vi "GetSettings.vi"(8 "error in (no error)":errorcluster, 10 "SettingsToRetrieve":variant, 11 "NHRDCPower in":refnum<class "NHRDCPower.lvclass">) -> (0 "error out":errorcluster, 1 "DeviceConfig&Meas":variant, 2 "RetrievedSettings":variant, 3 "NHRDCPower Out":refnum<class "NHRDCPower.lvclass">)   [LabVIEW 2018, in "AcPwrPlugins.lvlib" / "NHRDCPower.lvclass"]
doc: "This VI retrieves the configuration or measurement settings."
uses:
  NHRDCPower.lvclass
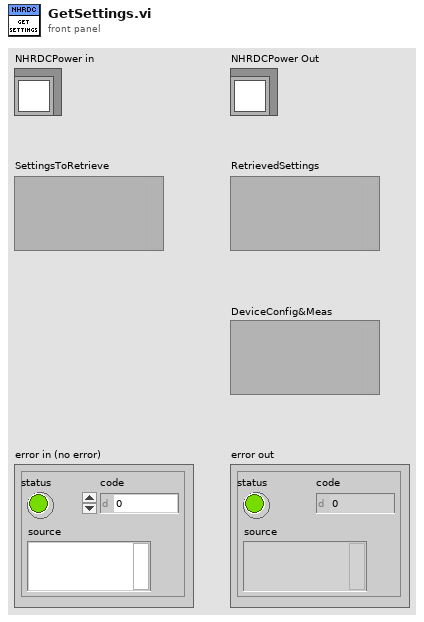
[diagram p1: front panel]
types:
  T1 = typedef "AcPwrPlugins.lvlib/NHRDCPower.lvclass/Device(s)Settings.ctl" = cluster{"MeasName":string, "Modules":T2}
  T2 = typedef "AcPwrPlugins.lvlib/NHRDCPower.lvclass/Modules.ctl" = cluster{"Handle":string, "Name":string, "id query (Yes)":bool, "reset device (Yes)":bool, "Connected":bool, "Initial Battery Detect Voltage (0)":dbl, "SafetySettings":cluster{"SetWatchDog?":bool, "Voltage (V)":dbl, "Current (A)":dbl, "Power (W)":dbl, "Voltage Delay (s)":dbl, "Current Delay (s)":dbl, "Power Delay (s)":dbl}, "Options String":string, "Aperture Time (s)":dbl, "operating state (Off)":i32, "OutputSettings":cluster{"Voltage (V)":dbl, "Current (A)":dbl, "Resistance (Ohms)":dbl, "Power (W)":dbl, "Enable Voltage":bool, "Enable Current":bool, "Enable Resistance":bool, "Enable Power":bool, "Macro After Step Delay  (s)":dbl, "Wait Value (V, A, W)":dbl, "Enable Wait":bool, "Wait on Value":i32}[], "SlewRate":cluster{"Set Voltage Rate V/S":dbl, "Set Current Rate A/S":dbl, "Set Resistance Rate R/S":dbl, "Set Power Rate W/S":dbl}, "Macro":cluster{"Save Macro?":bool, "Load Macro From File?":bool, "Run Macro Continuously?":bool, "Use Macros?":bool, "Load Macro File Path":string, "Save Macro File Path":string}, "Regulation Gain (1=100%)":dbl, "UpdatingOntheFly":bool}[]
  T3 = typedef "AcPwrPlugins.lvlib/NHRDCPower.lvclass/Measurements.ctl" = cluster{"Handle":string, "Name":string, "Enabled":bool, "Measurement Value":sgl, "Measurement Type":enum16{"Power", "Current", "Voltage"}}[]
  T4 = cluster{"xml string":string, "xml string":string}
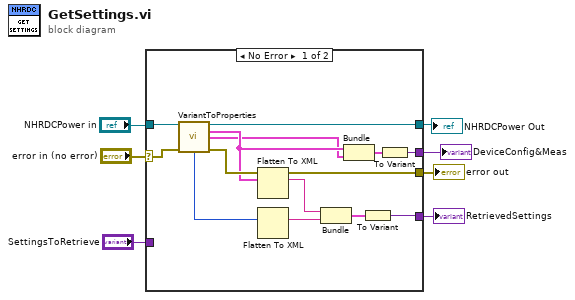
[diagram p0: block diagram]
diagram:
  n1 = case shown="No Error" "error in (no error)" {
    selector: "error in (no error)" -> [w20 w22]
    tunnel: "NHRDCPower in" -> [w19 w23]
    tunnel: [w18 w23] -> w6
    tunnel: [w17 w22] -> w5
    tunnel: "SettingsToRetrieve" -> [_ w21]
    tunnel: [w12 w21] -> w2
    tunnel: [w8 _] -> w1
    frame No Error {
      n2 = call "VariantToProperties.vi"("NHRDCPower in"=w19, "error in (no error)"=w20) -> ("NHRDCPower out"=w18:refnum<class "NHRDCPower.lvclass">, "NHRDC"=w11:T1, "Meas"=w10:T3, "Measurement Refresh Time (ms)"=w13:u32, "error out"=w17:errorcluster)  [unwired: 7 in, 2 out]
      n3 = Flatten To XML(anything=w11) -> (xml string=w15:string)
      n4 = Flatten To XML(anything=w13) -> (xml string=w14:string)
      n5 = Bundle("xml string"=w15, "xml string"=w14) -> (w16:T4)  [unwired: 1 in]
      n6 = Bundle("NHRDC"=w11, "Meas"=w10) -> (w9:cluster{"NHRDC":T1, "Meas":T3})  [unwired: 1 in]
      n7 = To Variant(anything=w16) -> (Variant=w12:variant)
      n8 = To Variant(anything=w9) -> (Variant=w8:variant)
    }
    frame Error {
    }
  }
  "error out" <- w5
  "NHRDCPower Out" <- w6
  "RetrievedSettings" <- w2
  "DeviceConfig&Meas" <- w1
